vi "Time-Delayed Send Message Core.vi"(4 "Caller Info":cluster{"Clone Type":string, "Clone ID":string}, 6 "Message Priority (Normal)":T1=enum."Normal", 7 "How Many Copies (0 = infinite repeat)":u32, 8 "Time To Wait":i32=1000, 9 "Delivery Notifier":refnum<notifier>, 10 "Message":refnum<class "Message.lvclass">, 11 "Message Enqueuer":refnum<class "Message Enqueuer.lvclass">) -> ()   [LabVIEW 2017]
doc: "This VI forms the core processing loop for the time-delayed messages. This VI may be called directly if the desired behavior is for the caller to wait until the messages have been sent before continuing, but the usual usage of this VI is to call <b>Time-Delayed Send Message.vi</b> which will launch an asynch clone of this VI so that the caller can proceed with other work instead of waiting for the time out. \n\nSee Context Help for <b>Time-Delayed Send Message.vi</b> for further details."
uses:
  <vilib>/ActorFramework/Message Enqueuer/Message Enqueuer.lvclass
  <vilib>/ActorFramework/Message/Message.lvclass
  <vilib>/ActorFramework/Time-Delayed Send Message/Time-Delay Override Options.ctl
  <vilib>/ActorFramework/Message Enqueuer/Message Priority.ctl
  <vilib>/ActorFramework/Message Enqueuer/Message Enqueuer.lvclass/Message Enqueuer.ctl
  <vilib>/ActorFramework/Message Priority Queue/Priority Enqueue.vi
  <resource>/AFDebug/AF Debug.lvlib
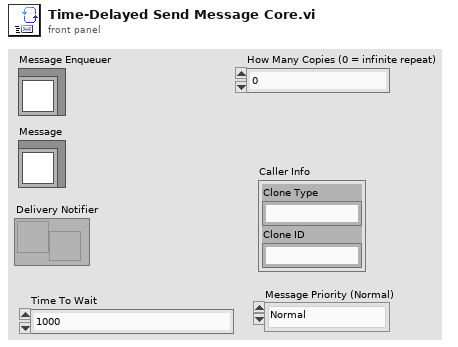
[diagram p1: front panel]
types:
  T1 = typedef "Actor Framework.lvlib/Message Enqueuer.lvclass/Message Priority.ctl" = enum16{"Low", "Normal", "High"}
  T2 = typedef "Time-Delay Override Options.ctl" = enum16{"Send next copy now", "Skip next scheduled copy", "Send next copy now and stop all further copies", "Stop all further copies"}
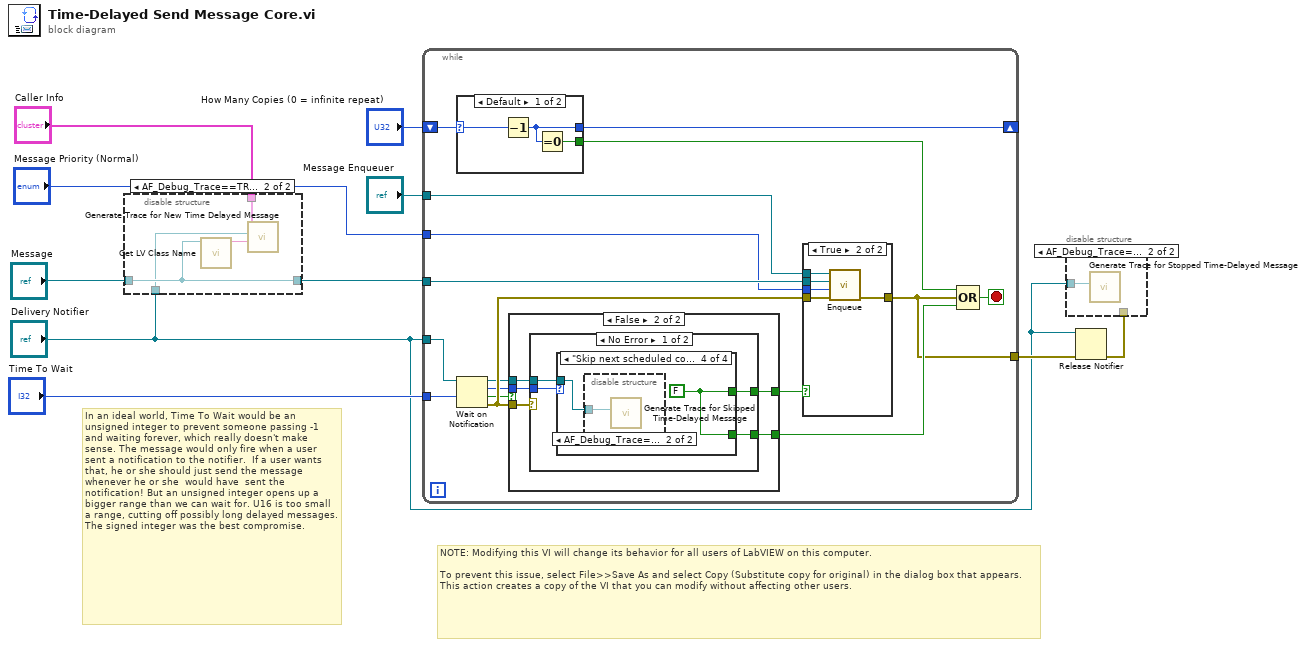
[diagram p0: block diagram]
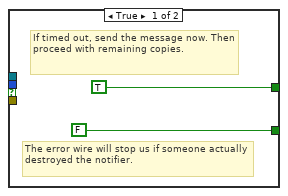
[diagram p4: hidden frame]
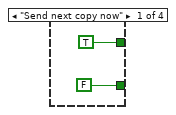
[diagram p5: hidden frame]
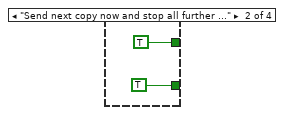
[diagram p6: hidden frame]
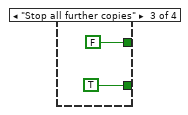
[diagram p7: hidden frame]
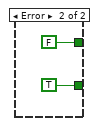
[diagram p9: hidden frame]
diagram:
  # "NOTE: Modifying this VI will change its behavior for all users of LabVIEW on this computer.\n\nTo prevent this issue, select File>>Save As and select Copy (Substitute copy for original) in the dialog box that appears. This action creates a copy of the VI that you can modify without affecting other users."
  # "In an ideal world, Time To Wait would be an unsigned integer to prevent someone passing -1 and waiting forever, which really doesn't make sense. The message would only fire when a user sent a notification to the notifier.  If a user wants that, he or she should just send the message whenever he or she  would have  sent the notification! But an unsigned integer opens up a bigger range than we can wait for. U16 is too small a range, cutting off possibly long delayed messages. The signed integer was the best compromise."
  n1 = disable-structure shown="AF_Debug_Trace==TRUE" {
    disable-tunnel: "Message" -> [w11 w14]
    disable-tunnel: [w11 w14] -> w4
    disable-tunnel: "Delivery Notifier" -> [_ w13]
    disable-tunnel: "Caller Info" -> [_ w12]
    frame condition #0 (active) {
    }
    frame condition #1 {
      n2 = call <vilib>:"Get LV Class Name.vi"("object"=w14) -> ("class name"=w15:string)  [unwired: 9 in, 1 out]
      n3 = call <resource>:"Generate Trace for New Time Delayed Message.vi"("Message Name"=w15, "Delivery Notifier"=w13, "Caller Details"=w12) -> ()  [unwired: 9 in]
    }
  }
  n4 = while {
    shift-right: [w29] -> _
    shift-left: "How Many Copies (0 = infinite repeat)" -> [w30]
    tunnel: "Delivery Notifier" -> [w28]
    tunnel: "Message Enqueuer" -> [w27]
    tunnel: w4 -> [w26]
    tunnel: "Time To Wait" -> [w20]
    tunnel: [w18] -> w7
    tunnel: "Message Priority (Normal)" -> [w17]
    stop <- w25 stop-if-true
    n5 = case shown="Default" w30 {
      selector: w30 -> [w62 w63]
      tunnel: [w61 w63] -> w29
      tunnel: [w60 _] -> w24
      frame Default {
        n6 = Decrement(x=w62) -> (x-1=w61:u32)
        n7 = Equal To 0?(x=w61) -> (x = 0?=w60:bool)
      }
      frame 0 {
      }
    }
    n8 = Wait on Notification(notifier=w28, timeout in ms (-1)=w20) -> (notifier out=w16:refnum<notifier>, notification=w21:T2, timed out?=w23:bool, error out=w31:errorcluster)  [unwired: 2 in]
    n9 = case shown="False" w23 {
      tunnel: [TRUE w37] -> w22
      tunnel: w21 -> [_ w36]
      tunnel: w31 -> [_ w38]
      tunnel: [FALSE w35] -> w19
      tunnel: w16 -> [_ w34]
      frame True {
        # "The error wire will stop us if someone actually destroyed the notifier."
        # "If timed out, send the message now. Then proceed with remaining copies."
      }
      frame False {
        n10 = case shown="No Error" w38 {
          tunnel: [w41 FALSE] -> w37
          tunnel: w36 -> [w42 _]
          tunnel: [w40 TRUE] -> w35
          tunnel: w34 -> [w39 _]
          frame No Error {
            n11 = case shown="\"Skip next scheduled copy\"" w42 {
              tunnel: [TRUE TRUE FALSE w50] -> w41
              tunnel: [FALSE TRUE TRUE w50] -> w40
              tunnel: w39 -> [_ _ _ w49]
              frame "Send next copy now" {
              }
              frame "Send next copy now and stop all further copies" {
              }
              frame "Stop all further copies" {
              }
              frame "Skip next scheduled copy" {
                w50 = FALSE
                n12 = disable-structure shown="AF_Debug_Trace==TRUE" {
                  disable-tunnel: w49 -> [_ w51]
                  frame condition #0 (active) {
                  }
                  frame condition #1 {
                    n13 = call <resource>:"Generate Trace for Skipped Time-Delayed Message.vi"("Delivery Notifier"=w51) -> ()  [unwired: 11 in]
                  }
                }
              }
            }
          }
          frame Error {
          }
        }
      }
    }
    n14 = case shown="True" w22 {
      tunnel: w27 -> [_ w59]
      tunnel: w26 -> [_ w58]
      tunnel: w31 -> [w54 w57]
      tunnel: [w54 w56] -> w18
      tunnel: w17 -> [_ w55]
      frame False {
      }
      frame True {
        n15 = call <vilib>:"Enqueue.vi"("error in (no error)"=w57, "Message Priority (Normal)"=w55, "Message"=w58, "Message Enqueuer in"=w59) -> ("error out"=w56:errorcluster)  [unwired: 6 in, 1 out]
      }
    }
    n16 = Compound Arithmetic op=OR(w24, w18, w19) -> (w25:bool)
  }
  n17 = Release Notifier(notifier="Delivery Notifier", error in (no error)=w7) -> (error out=w1:errorcluster)  [unwired: 1 in, 2 out]
  n18 = disable-structure shown="AF_Debug_Trace==TRUE" {
    disable-tunnel: "Delivery Notifier" -> [_ w64]
    disable-tunnel: w1 -> [_ _]
    frame condition #0 (active) {
    }
    frame condition #1 {
      n19 = call <resource>:"Generate Trace for Stopped Time-Delayed Message.vi"("Delivery Notifier"=w64) -> ()  [unwired: 11 in]
    }
  }
